vi "ReadConfiguration.vi"(8 "error in (no error)":errorcluster, 11 "VI Path":path) -> (0 "error out":errorcluster, 3 "StandbyArray":dbl[](array[numeric]))   [LabVIEW 2014]
uses:
  SystemConfigure.ctl
  <vilib>/Utility/config.llb/Read Key (Double).vi
  <vilib>/Utility/config.llb/NI_LVConfig.lvlib
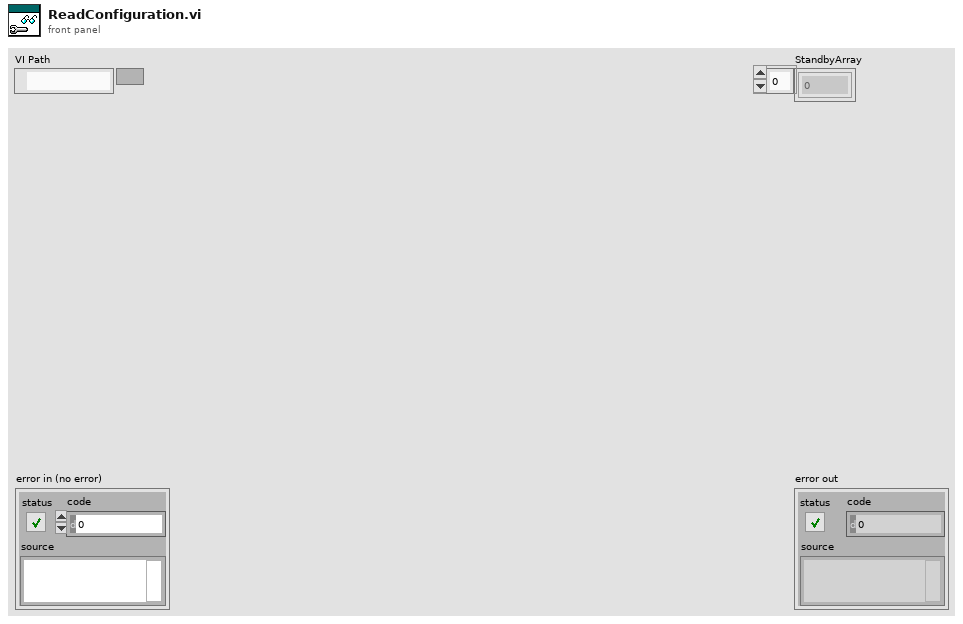
[diagram p1: front panel]
types:
  T1 = typedef "NI_LVConfig.lvlib/Config Data RefNum.ctl" = refnum<k1>
  T2 = typedef "SystemConfigure.ctl" = cluster{"DAQDevice":tag, "COMPort":refnum<visa-resource-name>, "Product":string}
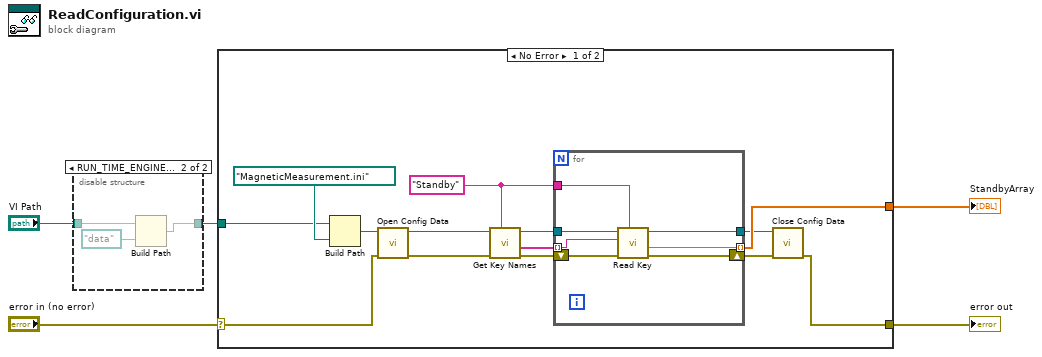
[diagram p0: block diagram]
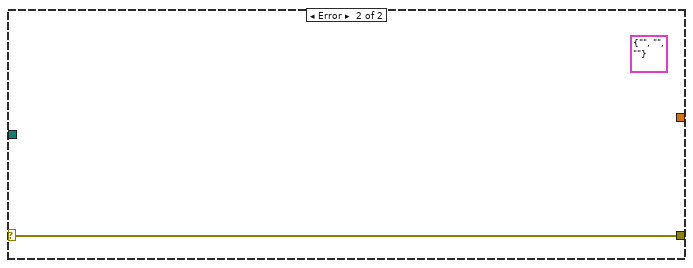
[diagram p3: hidden frame]
diagram:
  n1 = disable-structure shown="RUN_TIME_ENGINE==True" {
    disable-tunnel: "VI Path" -> [w6 w9]
    disable-tunnel: [w6 w8] -> w2
    frame condition #0 (active) {
    }
    frame condition #1 {
      n2 = Build Path(base path=w9, name or relative path=path "data") -> (appended path=w8:path)
    }
  }
  n3 = case shown="No Error" "error in (no error)" {
    selector: "error in (no error)" -> [w19 w31]
    tunnel: [w20 w31] -> w4
    tunnel: w2 -> [w21 _]
    tunnel: [w11 _] -> w1
    frame No Error {
      w17 = "Standby" ("section")
      n4 = Build Path(base path=w21, name or relative path=path "MagneticMeasurement.ini") -> (appended path=w23:path)
      n5 = call <vilib>:"Open Config Data.vi"("error in (no error)"=w19, "configuration file path"=w23) -> ("error out"=w12:errorcluster, "refnum"=w13:T1)  [unwired: 7 in, 1 out]
      n6 = call <vilib>:"Get Key Names.vi"("section"=w17, "error in (no error)"=w12, "refnum"=w13) -> ("error out"=w15:errorcluster, "key names"=w14:string[], "refnum out"=w18:T1)  [unwired: 5 in, 1 out]
      n7 = for {
        tunnel: w18 -> [w30]
        tunnel: w17 -> [w29]
        tunnel: [w28] -> w11 mode=indexing
        shift-right: [w27] -> w16
        shift-left: w15 -> [w26]
        tunnel: w14 -> [w25] mode=indexing
        tunnel: [w24] -> w10
        n8 = call-poly <vilib>:"Read Key.vi"("section"=w29, "error in (no error)"=w26, "key"=w25, "refnum"=w30) -> ("error out"=w27:errorcluster, "value"=w28:dbl, "refnum out"=w24:T1)  [unwired: 4 in, 1 out]
      }
      n9 = call <vilib>:"Close Config Data.vi"("error in (no error)"=w16, "refnum"=w10) -> ("error out"=w20:errorcluster)  [unwired: 8 in, 1 out]
    }
    frame Error {
      (unwired) T2 {"DAQDevice"="", "COMPort"="", "Product"=""} ("SystemConfigure")
    }
  }
  "error out" <- w4
  "StandbyArray" <- w1
